vi "CheckStepSetup.vi"(8 "error in (no error)":errorcluster, 11 "StepDataTable":string[](array[string])) -> (0 "error out":errorcluster, 2 "StepNames":cluster{string[]}[](array[cluster]), 3 "StepSetups":string[](array[string]))   [LabVIEW 2014, in "Project.lvclass"]
uses:
  Project.lvclass
  StepSetupDataTypeDefine.ctl
  StepData/Control/AllStepTypeData.ctl
  StepData/Control/StepTypeEnum.ctl
  StepData/Control/MoveData.ctl
  StepData/Control/MeasureData.ctl
  StepData/StepData.lvclass
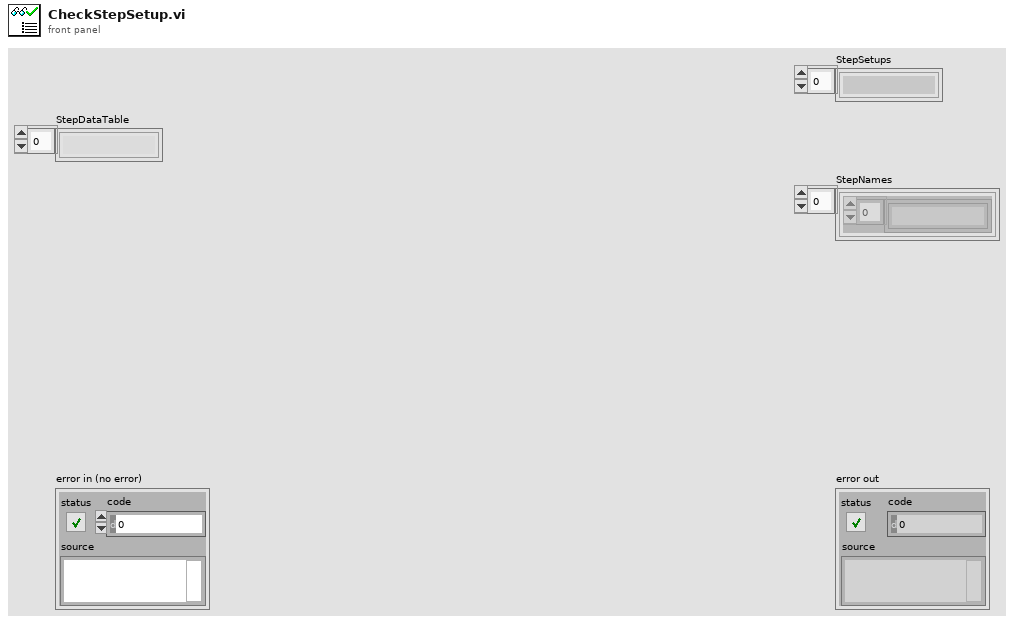
[diagram p1: front panel]
types:
  T1 = typedef "Project.lvclass/StepSetupDataTypeDefine.ctl" = cluster{"AllStepTypeData":T2}[]
  T2 = typedef "StepData.lvclass/AllStepTypeData.ctl" = cluster{"StepName":string, "StepTypeEnum":T3, "MoveData":T4, "MeasureData":T5}
  T3 = typedef "StepData.lvclass/StepTypeEnum.ctl" = enum16{"Move", "Measure"}
  T4 = typedef "StepData.lvclass/MoveData.ctl" = cluster{"Axis":u16, "Position":dbl, "Speed":dbl, "Acc/Dec":dbl, "Mode":u16}
  T5 = typedef "StepData.lvclass/MeasureData.ctl" = cluster{"Sensor No.":i32, "Log?":bool}
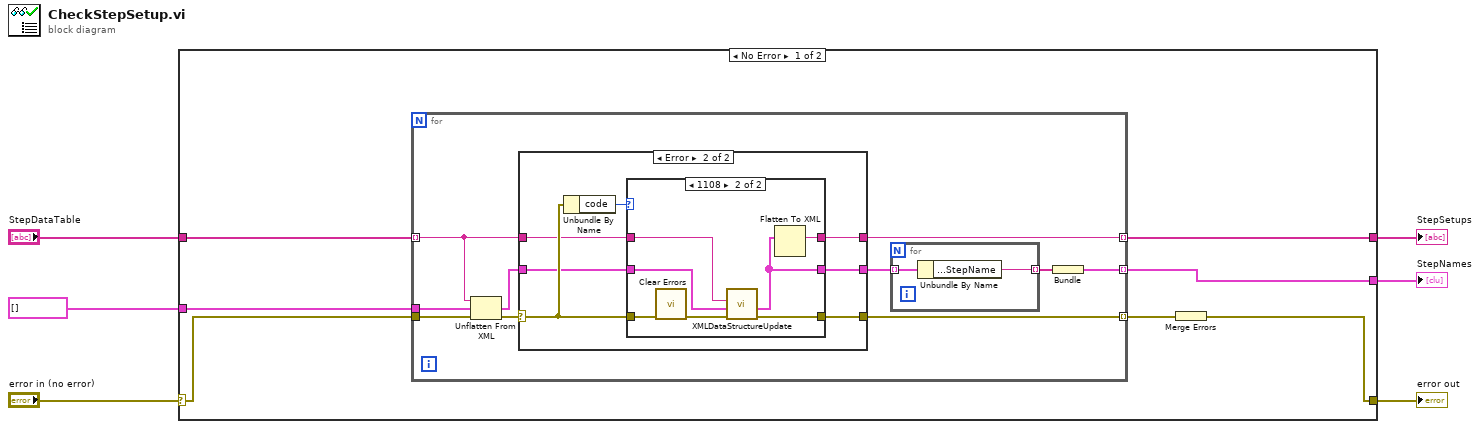
[diagram p0: block diagram]
diagram:
  n1 = case shown="No Error" "error in (no error)" {
    selector: "error in (no error)" -> [w13 w46]
    tunnel: [w10 w46] -> w5
    tunnel: T1 [] ("StepSetupClusterArray") -> [w12 _]
    tunnel: [w9 _] -> w3
    tunnel: "StepDataTable" -> [w8 _]
    tunnel: [w7 _] -> w1
    frame No Error {
      n2 = for {
        tunnel: w8 -> [w17] mode=indexing
        tunnel: w13 -> [w23]
        tunnel: [w20] -> w9 mode=indexing
        tunnel: w12 -> [w18]
        tunnel: [w16] -> w11 mode=indexing
        tunnel: [w14] -> w7 mode=indexing
        n3 = Unflatten From XML(xml string=w17, type=w18, error in (no error)=w23) -> (value=w21:T1, error out=w22:errorcluster)
        n4 = case shown="Error" w22 {
          selector: w22 -> [w28 w34]
          tunnel: w21 -> [w26 w33]
          tunnel: [w27 w32] -> w20
          tunnel: [w26 w31] -> w19
          tunnel: w17 -> [w27 w30]
          tunnel: [w28 w29] -> w16
          frame No Error {
          }
          frame Error {
            n5 = Unbundle By Name(w34) -> ("code"=w35:i32)
            n6 = case shown="1108" w35 {
              tunnel: w34 -> [w36 w45]
              tunnel: w33 -> [w37 w41]
              tunnel: [w38 w44] -> w32
              tunnel: [w37 w40] -> w31
              tunnel: w30 -> [w38 w43]
              tunnel: [w36 w39] -> w29
              frame Default {
              }
              frame 1108 {
                n7 = call <vilib>:"Clear Errors.vi"("error in (no error)"=w45) -> ("error out"=w42:errorcluster)  [unwired: 5 in, 1 out]
                n8 = call "XMLDataStructureUpdate.vi"("error in (no error)"=w42, "NewType In"=w41, "XMLString In"=w43) -> ("error out"=w39:errorcluster, "NewType Out"=w40:T1)  [unwired: 7 in]
                n9 = Flatten To XML(anything=w40) -> (xml string=w44:string)
              }
            }
          }
        }
        n10 = for {
          tunnel: w19 -> [w25] mode=indexing
          tunnel: [w24] -> w15 mode=indexing
          n11 = Unbundle By Name(w25) -> ("AllStepTypeData.StepName"=w24:string)
        }
        n12 = Bundle(w15) -> (w14:cluster{string[]})  [unwired: 1 in]
      }
      n13 = Merge Errors(w11) -> (w10:errorcluster)
    }
    frame Error {
    }
  }
  "error out" <- w5
  "StepSetups" <- w3
  "StepNames" <- w1
